vi "PH_AxisGUI_BaseClass.PC Absolute Move.vi"(0 "i ref in":refnum<vi>, 2 "Axis":i32=-1, 4 "Position [Units]":dbl, 5 "error in":errorcluster) -> (14 "i ref out":refnum<vi>, 19 "error out":errorcluster)   [LabVIEW 2014, in "PH_AxisGUI_BaseClass.lvlib"]
doc: "This VI acts on an axis."
uses:
  PH_AxisGUI_BaseClass.lvlib
  PH_Stepmotor_BaseClass/PH_Stepmotor_BaseClass.lvlib
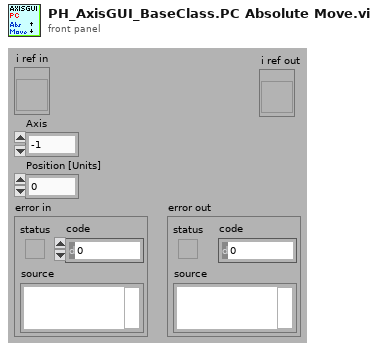
[diagram p1: front panel]
types:
  T1 = typedef "PH_Stepmotor_BaseClass.lvlib/PH_Stepmotor_BaseClass.Axis Address.ctl" = cluster{"Instance":string, "Motor Nr":i32}
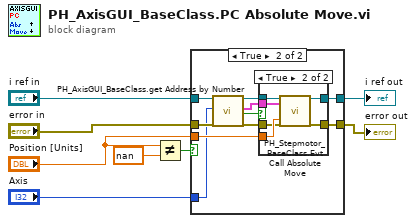
[diagram p0: block diagram]
diagram:
  n1 = Not Equal?(x="Position [Units]", y=nan) -> (x != y?=w1:bool)
  n2 = case shown="True" w1 {
    tunnel: "Position [Units]" -> [_ w18]
    tunnel: "i ref in" -> [w10 w17]
    tunnel: "error in" -> [w9 w16]
    tunnel: [w10 w15] -> w6
    tunnel: [w9 w14] -> w5
    tunnel: "Axis" -> [_ w11]
    frame False {
    }
    frame True {
      n3 = call "PH_AxisGUI_BaseClass.get Address by Number.vi"("VI in"=w17, "Axis"=w11, "error in (no error)"=w16) -> ("VI out"=w20:refnum<vi>, "Address"=w13:T1, "Axis exists and is not moving?"=w12:bool, "error out"=w19:errorcluster)  [unwired: 12 in, 1 out]
      n4 = case "Axis moving or no motion instance?" shown="True" w12 {
        tunnel: w18 -> [_ w28]
        tunnel: [w22 w23] -> w15
        tunnel: [w21 w24] -> w14
        tunnel: w20 -> [w22 w27]
        tunnel: w19 -> [w21 w26]
        tunnel: w13 -> [_ w25]
        frame False {
        }
        frame True {
          n5 = call "PH_Stepmotor_BaseClass.Evt Call Absolute Move.vi"("i ref in"=w27, "Address"=w25, "error in"=w26, "Target Position (Units)"=w28) -> ("i ref out"=w23:refnum<vi>, "error out"=w24:errorcluster)  [unwired: 14 in]
        }
      }
    }
  }
  "error out" <- w5
  "i ref out" <- w6
